vi "ScaleJS.vi"(8 "Buttons":bool[](array[boolean]), 11 "Axis In":dbl) -> (3 "Axis Out":dbl)   [LabVIEW 2014]
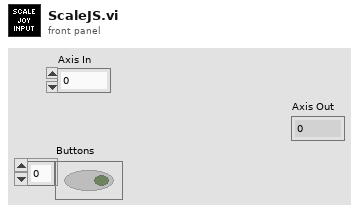
[diagram p1: front panel]
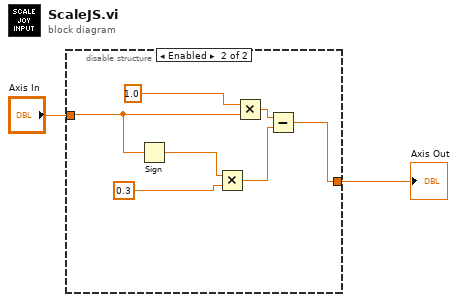
[diagram p0: block diagram]
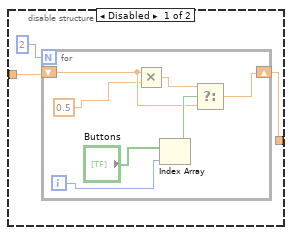
[diagram p2: hidden frame]
diagram:
  n1 = disable-structure shown="Enabled" {
    disable-tunnel: "Axis In" -> [w4 w16]
    disable-tunnel: [w3 w13] -> w1
    frame Disabled {
      n2 = for {
        N: 2 -> [_]
        shift-right: [w7] -> w3
        shift-left: w4 -> [w8]
        i -> [w10]
        n3 = Multiply(x=w8, y=0.5) -> (x*y=w9:dbl)
        n4 = Index Array(array="Buttons", index=w10) -> (element=w11:bool)
        n5 = Select(t=w9, s=w11, f=w8) -> (s? t:f=w7:dbl)
      }
    }
    frame Enabled {
      n6 = Sign(1:w16) -> (0:w15:dbl)
      n7 = Multiply(x=w15, y=0.3) -> (x*y=w14:dbl)
      n8 = Multiply(x=1.0, y=w16) -> (x*y=w18:dbl)
      n9 = Subtract(x=w18, y=w14) -> (x-y=w13:dbl)
    }
  }
  "Axis Out" <- w1
